vi "To Serial Form.vi"(8 "error in (no error)":errorcluster, 9 "Metadata":variant, 10 "CI Serializer in":refnum<class "CI Serializer.lvclass">, 11 "Serializable Node in":refnum<class "Serializable Node.lvclass">) -> (0 "error out":errorcluster, 1 "Serialized Job Name":string, 2 "CI Serializer out":refnum<class "CI Serializer.lvclass">, 3 "Serializable Node out":refnum<class "Serializable Node.lvclass">)   [LabVIEW 2014, in "Serializable Node.lvclass"]
uses:
  Serializable Node.lvclass
  CI Serializer/CI Serializer.lvclass
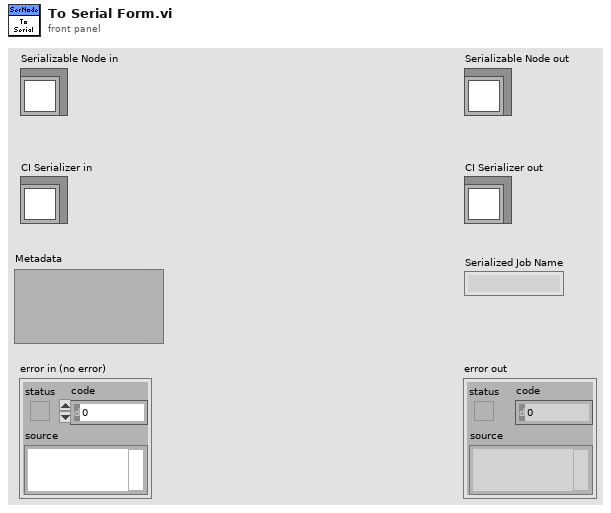
[diagram p1: front panel]
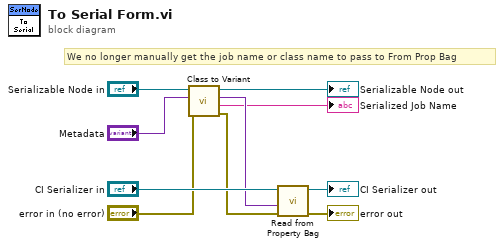
[diagram p0: block diagram]
diagram:
  # "We no longer manually get the job name or class name to pass to From Prop Bag"
  n1 = call-dynamic "Class to Variant.vi"("error in (no error)"="error in (no error)", "Data in"="Metadata", "Serializable Node in"="Serializable Node in") -> ("error out"=w4:errorcluster, "Serialized Object Name"=→"Serialized Job Name":string, "Data Out"=w5:variant, "Serializable Node out"=→"Serializable Node out":refnum<class "Serializable Node.lvclass">)  [unwired: 5 in]
  n2 = call-dynamic "Read from Property Bag.vi"("error in (no error)"=w4, "Data in"=w5, "CI Serializer in"="CI Serializer in") -> ("error out"=→"error out":errorcluster, "CI Serializer out"=→"CI Serializer out":refnum<class "CI Serializer.lvclass">)  [unwired: 7 in]
